vi "datatojson.vi"() -> (3 "json":string[](array[string]))   [LabVIEW 2022 SP3, in "工况数据上传.lvlib"]
panel:
  out "data":T1={"time"="2021-05-08 14-02-02", "data"={"ups"={"ups"={"input_voltage"=0.0, "input_frequency"=0.0, "output_voltage"=0.0, "output_current"=0.0, "output_frequency"=0.0, "output_active_power"=0.0, "output_apparent_power"=0.0, "load_rate"=0.0, "cabinet_temperature"=0.0, "battery_voltage"=0.0, "remaining_battery_capacity"=0.0, "power_on_status"="", "power_supply_mode"="", "fault"=FALSE, "battery_low_voltage"=FALSE, "mains_supply_abnormality"=FALSE}, "启用"=FALSE}, "air_conditioner"={"air_conditioner"={"cabinet_temperature"=0.0, "air_supply_temperature"=0.0, "voltage"=0.0, "current"=0.0, "compressor_status"="", "Internal_fan_status"="", "external_fan_status"="", "heating_state"="", "refrigeration_state"=FALSE, "high_temperature_alarm"=FALSE, "low_temperature_alarm"=FALSE, "heater_fault"=FALSE, "temperature_sensor_fault"=FALSE, "high_voltage_alarm"=FALSE, "low_voltage_alarm"=FALSE, "refrigeration_start_point"=0.0, "refrigeration_sensitive_point"=0.0, "heating_start_point"=0.0, "heating_sensitive_point"=0.0, "high_temperature_alarm_point"=0.0, "low_temperature_alarm_point"=0.0}, "启用"=FALSE}, "smoke_sensor"={"smoke_sensor"={"trigger_alarm"=FALSE}, "启用"=FALSE}, "water_immersion_sensor"={"water_immersion_sensor"={"trigger_alarm"=FALSE}, "启用"=FALSE}, "temperature_and_humidity_sensor"={"temperature_and_humidity_sensor"={"current_temperature"=0.0, "current_humidity"=0.0, "room_temperature_alarm"=FALSE, "humidity_alarm"=FALSE}, "启用"=FALSE}, "gps"={"gps"={"current_longitude"=0.0, "current_latitude"=0.0, "launch_longitude"=0.0, "launch_latitude"=0.0, "shift_alarm"=FALSE}, "启用"=FALSE}, "solar_controller"={"solar_controller"={"array_voltage"=0.0, "array_current"=0.0, "generating_power"=0.0, "battery_voltage"=0.0, "battery_current"=0.0, "ceiling_voltage"=0.0, "minimum_voltage"=0.0, "battery_temperature"=0.0, "remaining_battery_capacity"=0.0, "load_voltage"=0.0, "load_current"=0.0, "load_power"=0.0, "equipment_temperature"=0.0, "accumulated_electricity_consumption_of_the_day"=0.0, "accumulated_electricity_consumption_of_the_current_month"=0.0, "accumulated_electricity_consumption_in_the_current_year"=0.0, "total_accumulated_power_consumption"=0.0, "accumulated_charging_capacity_of_the_day"=0.0, "accumulated_charging_amount_of_the_current_month"=0.0, "accumulated_charging_capacity_of_the_current_year"=0.0, "total_cumulative_charge"=0.0}, "启用"=FALSE}, "solar_controller_2"={"solar_controller_2"={"array_voltage"=0.0, "array_current"=0.0, "generating_power"=0.0, "battery_voltage"=0.0, "battery_current"=0.0, "ceiling_voltage"=0.0, "minimum_voltage"=0.0, "battery_temperature"=0.0, "remaining_battery_capacity"=0.0, "load_voltage"=0.0, "load_current"=0.0, "load_power"=0.0, "equipment_temperature"=0.0, "accumulated_electricity_consumption_of_the_day"=0.0, "accumulated_electricity_consumption_of_the_current_month"=0.0, "accumulated_electricity_consumption_in_the_current_year"=0.0, "total_accumulated_power_consumption"=0.0, "accumulated_charging_capacity_of_the_day"=0.0, "accumulated_charging_amount_of_the_current_month"=0.0, "accumulated_charging_capacity_of_the_current_year"=0.0, "total_cumulative_charge"=0.0}, "启用"=FALSE}, "NH3"={"NH3"={"F0"=0.0, "F1"=0.0, "syringe_temperature"=0.0, "alarm_step"=0.0, "X0"=0.0}, "启用"=FALSE}, "TP"={"TP"={"F0"=0.0, "F1"=0.0, "F2"=0.0, "F3"=0.0, "digestion_temperature"=0.0, "constant_temperature"=0.0, "syringe_temperature"=0.0, "alarm_step"=0.0, "X0"=0.0}, "启用"=FALSE}, "TN"={"TN"={"F0"=0.0, "F1"=0.0, "F2"=0.0, "F3"=0.0, "F4"=0.0, "F5"=0.0, "F6"=0.0, "F7"=0.0, "digestion_temperature"=0.0, "constant_temperature"=0.0, "syringe_temperature"=0.0, "alarm_step"=0.0, "X0"=0.0}, "启用"=FALSE}, "CODMn"={"CODMn"={"temperature_curve"=[], "titration_curve"=[], "F0"=0.0, "F1"=0.0, "F2"=0.0, "F3"=0.0, "F4"=0.0, "F5"=0.0, "A"=0.0, "B"=0.0, "K"=0.0}, "启用"=FALSE}, "CODCr"={"CODCr"={"temperature_curve"=[], "F0"=0.0, "F1"=0.0, "reagent_sensor"=0.0}, "启用"=FALSE}}} {"data"."air_conditioner"."air_conditioner"."current" format="%#.2g"}
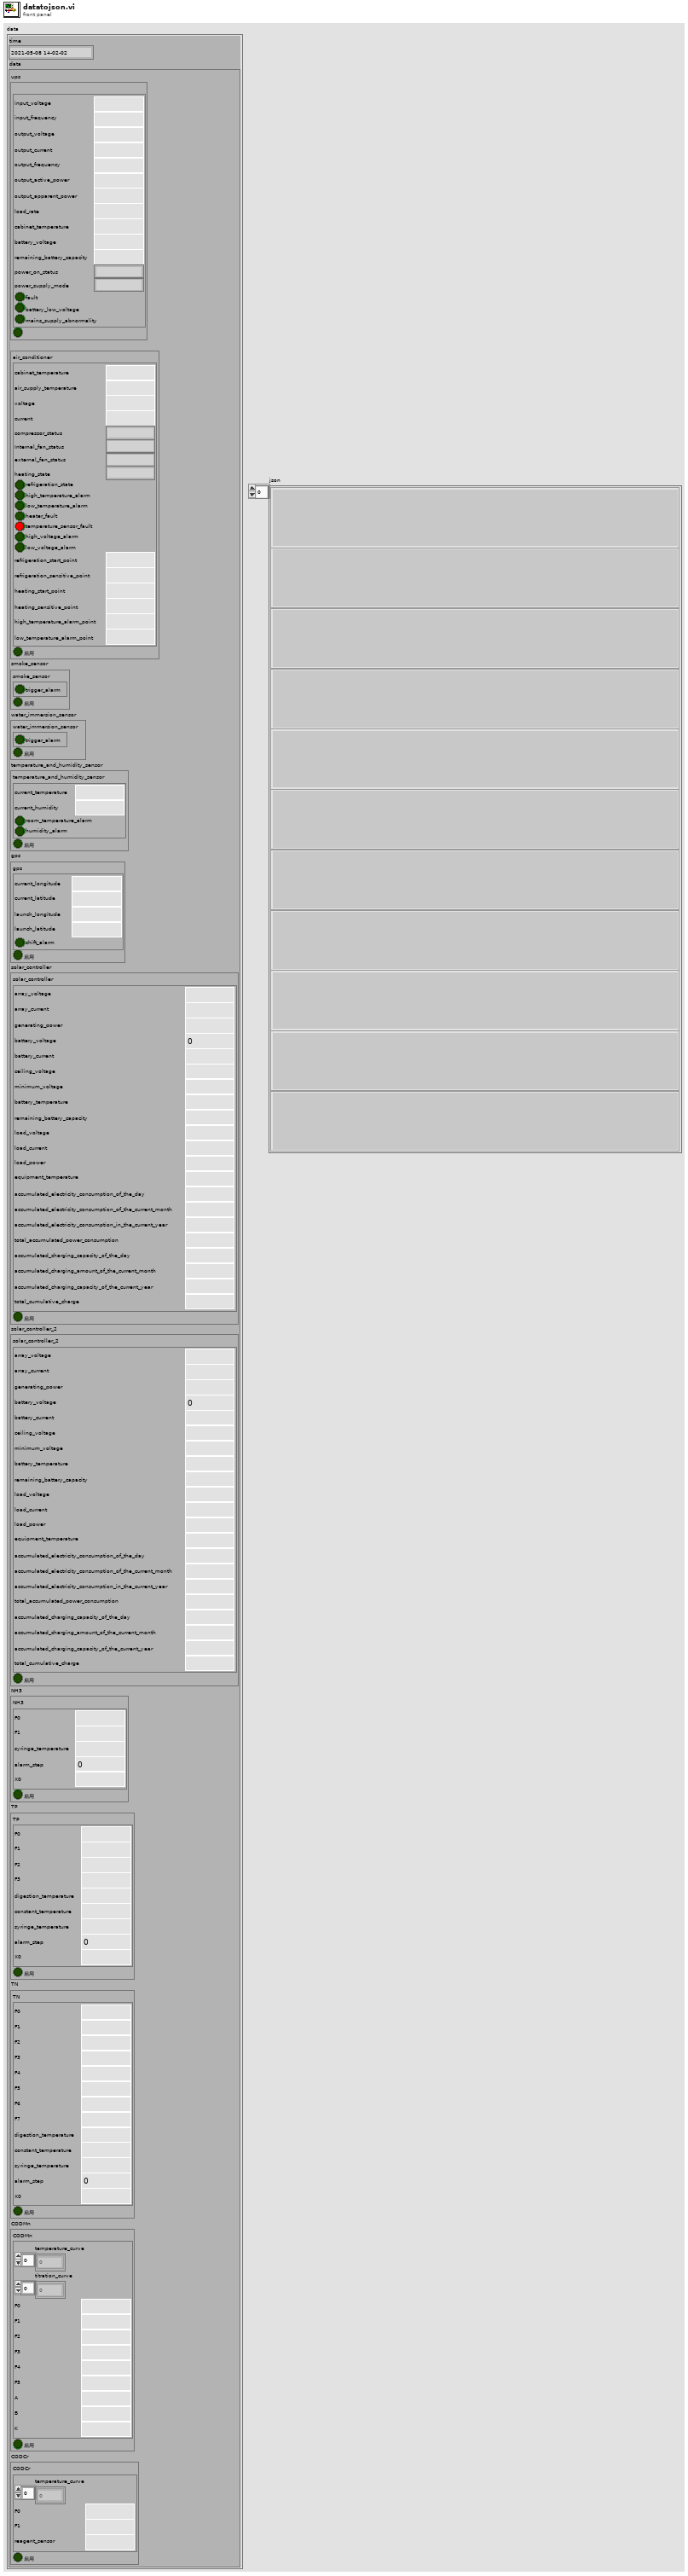
[diagram p1: front panel]
types:
  T1 = typedef "工况数据.ctl" = cluster{"time":string, "data":cluster{"ups":cluster{"ups":cluster{"input_voltage":ext, "input_frequency":ext, "output_voltage":ext, "output_current":ext, "output_frequency":ext, "output_active_power":ext, "output_apparent_power":ext, "load_rate":ext, "cabinet_temperature":ext, "battery_voltage":ext, "remaining_battery_capacity":ext, "power_on_status":string, "power_supply_mode":string, "fault":bool, "battery_low_voltage":bool, "mains_supply_abnormality":bool}, "启用":bool}, "air_conditioner":cluster{"air_conditioner":cluster{"cabinet_temperature":ext, "air_supply_temperature":ext, "voltage":ext, "current":ext, "compressor_status":string, "Internal_fan_status":string, "external_fan_status":string, "heating_state":string, "refrigeration_state":bool, "high_temperature_alarm":bool, "low_temperature_alarm":bool, "heater_fault":bool, "temperature_sensor_fault":bool, "high_voltage_alarm":bool, "low_voltage_alarm":bool, "refrigeration_start_point":ext, "refrigeration_sensitive_point":ext, "heating_start_point":ext, "heating_sensitive_point":ext, "high_temperature_alarm_point":ext, "low_temperature_alarm_point":ext}, "启用":bool}, "smoke_sensor":cluster{"smoke_sensor":cluster{"trigger_alarm":bool}, "启用":bool}, "water_immersion_sensor":cluster{"water_immersion_sensor":cluster{"trigger_alarm":bool}, "启用":bool}, "temperature_and_humidity_sensor":cluster{"temperature_and_humidity_sensor":cluster{"current_temperature":ext, "current_humidity":ext, "room_temperature_alarm":bool, "humidity_alarm":bool}, "启用":bool}, "gps":cluster{"gps":cluster{"current_longitude":ext, "current_latitude":ext, "launch_longitude":ext, "launch_latitude":ext, "shift_alarm":bool}, "启用":bool}, "solar_controller":cluster{"solar_controller":cluster{"array_voltage":ext, "array_current":ext, "generating_power":ext, "battery_voltage":dbl, "battery_current":ext, "ceiling_voltage":ext, "minimum_voltage":ext, "battery_temperature":ext, "remaining_battery_capacity":ext, "load_voltage":ext, "load_current":ext, "load_power":ext, "equipment_temperature":ext, "accumulated_electricity_consumption_of_the_day":ext, "accumulated_electricity_consumption_of_the_current_month":ext, "accumulated_electricity_consumption_in_the_current_year":ext, "total_accumulated_power_consumption":ext, "accumulated_charging_capacity_of_the_day":ext, "accumulated_charging_amount_of_the_current_month":ext, "accumulated_charging_capacity_of_the_current_year":ext, "total_cumulative_charge":ext}, "启用":bool}, "solar_controller_2":cluster{"solar_controller_2":cluster{"array_voltage":ext, "array_current":ext, "generating_power":ext, "battery_voltage":dbl, "battery_current":ext, "ceiling_voltage":ext, "minimum_voltage":ext, "battery_temperature":ext, "remaining_battery_capacity":ext, "load_voltage":ext, "load_current":ext, "load_power":ext, "equipment_temperature":ext, "accumulated_electricity_consumption_of_the_day":ext, "accumulated_electricity_consumption_of_the_current_month":ext, "accumulated_electricity_consumption_in_the_current_year":ext, "total_accumulated_power_consumption":ext, "accumulated_charging_capacity_of_the_day":ext, "accumulated_charging_amount_of_the_current_month":ext, "accumulated_charging_capacity_of_the_current_year":ext, "total_cumulative_charge":ext}, "启用":bool}, "NH3":cluster{"NH3":cluster{"F0":ext, "F1":ext, "syringe_temperature":ext, "alarm_step":dbl, "X0":ext}, "启用":bool}, "TP":cluster{"TP":cluster{"F0":ext, "F1":ext, "F2":ext, "F3":ext, "digestion_temperature":ext, "constant_temperature":ext, "syringe_temperature":ext, "alarm_step":dbl, "X0":ext}, "启用":bool}, "TN":cluster{"TN":cluster{"F0":ext, "F1":ext, "F2":ext, "F3":ext, "F4":ext, "F5":ext, "F6":ext, "F7":ext, "digestion_temperature":ext, "constant_temperature":ext, "syringe_temperature":ext, "alarm_step":dbl, "X0":ext}, "启用":bool}, "CODMn":cluster{"CODMn":cluster{"temperature_curve":ext[], "titration_curve":ext[], "F0":ext, "F1":ext, "F2":ext, "F3":ext, "F4":ext, "F5":ext, "A":ext, "B":ext, "K":ext}, "启用":bool}, "CODCr":cluster{"CODCr":cluster{"temperature_curve":ext[], "F0":ext, "F1":ext, "reagent_sensor":ext}, "启用":bool}}}
  T2 = cluster{"ups":cluster{"ups":cluster{"input_voltage":ext, "input_frequency":ext, "output_voltage":ext, "output_current":ext, "output_frequency":ext, "output_active_power":ext, "output_apparent_power":ext, "load_rate":ext, "cabinet_temperature":ext, "battery_voltage":ext, "remaining_battery_capacity":ext, "power_on_status":string, "power_supply_mode":string, "fault":bool, "battery_low_voltage":bool, "mains_supply_abnormality":bool}, "启用":bool}, "air_conditioner":cluster{"air_conditioner":cluster{"cabinet_temperature":ext, "air_supply_temperature":ext, "voltage":ext, "current":ext, "compressor_status":string, "Internal_fan_status":string, "external_fan_status":string, "heating_state":string, "refrigeration_state":bool, "high_temperature_alarm":bool, "low_temperature_alarm":bool, "heater_fault":bool, "temperature_sensor_fault":bool, "high_voltage_alarm":bool, "low_voltage_alarm":bool, "refrigeration_start_point":ext, "refrigeration_sensitive_point":ext, "heating_start_point":ext, "heating_sensitive_point":ext, "high_temperature_alarm_point":ext, "low_temperature_alarm_point":ext}, "启用":bool}, "smoke_sensor":cluster{"smoke_sensor":cluster{"trigger_alarm":bool}, "启用":bool}, "water_immersion_sensor":cluster{"water_immersion_sensor":cluster{"trigger_alarm":bool}, "启用":bool}, "temperature_and_humidity_sensor":cluster{"temperature_and_humidity_sensor":cluster{"current_temperature":ext, "current_humidity":ext, "room_temperature_alarm":bool, "humidity_alarm":bool}, "启用":bool}, "gps":cluster{"gps":cluster{"current_longitude":ext, "current_latitude":ext, "launch_longitude":ext, "launch_latitude":ext, "shift_alarm":bool}, "启用":bool}, "solar_controller":cluster{"solar_controller":cluster{"array_voltage":ext, "array_current":ext, "generating_power":ext, "battery_voltage":dbl, "battery_current":ext, "ceiling_voltage":ext, "minimum_voltage":ext, "battery_temperature":ext, "remaining_battery_capacity":ext, "load_voltage":ext, "load_current":ext, "load_power":ext, "equipment_temperature":ext, "accumulated_electricity_consumption_of_the_day":ext, "accumulated_electricity_consumption_of_the_current_month":ext, "accumulated_electricity_consumption_in_the_current_year":ext, "total_accumulated_power_consumption":ext, "accumulated_charging_capacity_of_the_day":ext, "accumulated_charging_amount_of_the_current_month":ext, "accumulated_charging_capacity_of_the_current_year":ext, "total_cumulative_charge":ext}, "启用":bool}, "solar_controller_2":cluster{"solar_controller_2":cluster{"array_voltage":ext, "array_current":ext, "generating_power":ext, "battery_voltage":dbl, "battery_current":ext, "ceiling_voltage":ext, "minimum_voltage":ext, "battery_temperature":ext, "remaining_battery_capacity":ext, "load_voltage":ext, "load_current":ext, "load_power":ext, "equipment_temperature":ext, "accumulated_electricity_consumption_of_the_day":ext, "accumulated_electricity_consumption_of_the_current_month":ext, "accumulated_electricity_consumption_in_the_current_year":ext, "total_accumulated_power_consumption":ext, "accumulated_charging_capacity_of_the_day":ext, "accumulated_charging_amount_of_the_current_month":ext, "accumulated_charging_capacity_of_the_current_year":ext, "total_cumulative_charge":ext}, "启用":bool}, "NH3":cluster{"NH3":cluster{"F0":ext, "F1":ext, "syringe_temperature":ext, "alarm_step":dbl, "X0":ext}, "启用":bool}, "TP":cluster{"TP":cluster{"F0":ext, "F1":ext, "F2":ext, "F3":ext, "digestion_temperature":ext, "constant_temperature":ext, "syringe_temperature":ext, "alarm_step":dbl, "X0":ext}, "启用":bool}, "TN":cluster{"TN":cluster{"F0":ext, "F1":ext, "F2":ext, "F3":ext, "F4":ext, "F5":ext, "F6":ext, "F7":ext, "digestion_temperature":ext, "constant_temperature":ext, "syringe_temperature":ext, "alarm_step":dbl, "X0":ext}, "启用":bool}, "CODMn":cluster{"CODMn":cluster{"temperature_curve":ext[], "titration_curve":ext[], "F0":ext, "F1":ext, "F2":ext, "F3":ext, "F4":ext, "F5":ext, "A":ext, "B":ext, "K":ext}, "启用":bool}, "CODCr":cluster{"CODCr":cluster{"temperature_curve":ext[], "F0":ext, "F1":ext, "reagent_sensor":ext}, "启用":bool}}
  T3 = cluster{"ups":cluster{"input_voltage":ext, "input_frequency":ext, "output_voltage":ext, "output_current":ext, "output_frequency":ext, "output_active_power":ext, "output_apparent_power":ext, "load_rate":ext, "cabinet_temperature":ext, "battery_voltage":ext, "remaining_battery_capacity":ext, "power_on_status":string, "power_supply_mode":string, "fault":bool, "battery_low_voltage":bool, "mains_supply_abnormality":bool}, "启用":bool}
  T4 = cluster{"air_conditioner":cluster{"cabinet_temperature":ext, "air_supply_temperature":ext, "voltage":ext, "current":ext, "compressor_status":string, "Internal_fan_status":string, "external_fan_status":string, "heating_state":string, "refrigeration_state":bool, "high_temperature_alarm":bool, "low_temperature_alarm":bool, "heater_fault":bool, "temperature_sensor_fault":bool, "high_voltage_alarm":bool, "low_voltage_alarm":bool, "refrigeration_start_point":ext, "refrigeration_sensitive_point":ext, "heating_start_point":ext, "heating_sensitive_point":ext, "high_temperature_alarm_point":ext, "low_temperature_alarm_point":ext}, "启用":bool}
  T5 = cluster{"smoke_sensor":cluster{"trigger_alarm":bool}, "启用":bool}
  T6 = cluster{"water_immersion_sensor":cluster{"trigger_alarm":bool}, "启用":bool}
  T7 = cluster{"temperature_and_humidity_sensor":cluster{"current_temperature":ext, "current_humidity":ext, "room_temperature_alarm":bool, "humidity_alarm":bool}, "启用":bool}
  T8 = cluster{"gps":cluster{"current_longitude":ext, "current_latitude":ext, "launch_longitude":ext, "launch_latitude":ext, "shift_alarm":bool}, "启用":bool}
  T9 = cluster{"solar_controller":cluster{"array_voltage":ext, "array_current":ext, "generating_power":ext, "battery_voltage":dbl, "battery_current":ext, "ceiling_voltage":ext, "minimum_voltage":ext, "battery_temperature":ext, "remaining_battery_capacity":ext, "load_voltage":ext, "load_current":ext, "load_power":ext, "equipment_temperature":ext, "accumulated_electricity_consumption_of_the_day":ext, "accumulated_electricity_consumption_of_the_current_month":ext, "accumulated_electricity_consumption_in_the_current_year":ext, "total_accumulated_power_consumption":ext, "accumulated_charging_capacity_of_the_day":ext, "accumulated_charging_amount_of_the_current_month":ext, "accumulated_charging_capacity_of_the_current_year":ext, "total_cumulative_charge":ext}, "启用":bool}
  T10 = cluster{"solar_controller_2":cluster{"array_voltage":ext, "array_current":ext, "generating_power":ext, "battery_voltage":dbl, "battery_current":ext, "ceiling_voltage":ext, "minimum_voltage":ext, "battery_temperature":ext, "remaining_battery_capacity":ext, "load_voltage":ext, "load_current":ext, "load_power":ext, "equipment_temperature":ext, "accumulated_electricity_consumption_of_the_day":ext, "accumulated_electricity_consumption_of_the_current_month":ext, "accumulated_electricity_consumption_in_the_current_year":ext, "total_accumulated_power_consumption":ext, "accumulated_charging_capacity_of_the_day":ext, "accumulated_charging_amount_of_the_current_month":ext, "accumulated_charging_capacity_of_the_current_year":ext, "total_cumulative_charge":ext}, "启用":bool}
  T11 = cluster{"NH3":cluster{"F0":ext, "F1":ext, "syringe_temperature":ext, "alarm_step":dbl, "X0":ext}, "启用":bool}
  T12 = cluster{"TP":cluster{"F0":ext, "F1":ext, "F2":ext, "F3":ext, "digestion_temperature":ext, "constant_temperature":ext, "syringe_temperature":ext, "alarm_step":dbl, "X0":ext}, "启用":bool}
  T13 = cluster{"TN":cluster{"F0":ext, "F1":ext, "F2":ext, "F3":ext, "F4":ext, "F5":ext, "F6":ext, "F7":ext, "digestion_temperature":ext, "constant_temperature":ext, "syringe_temperature":ext, "alarm_step":dbl, "X0":ext}, "启用":bool}
  T14 = cluster{"CODMn":cluster{"temperature_curve":ext[], "titration_curve":ext[], "F0":ext, "F1":ext, "F2":ext, "F3":ext, "F4":ext, "F5":ext, "A":ext, "B":ext, "K":ext}, "启用":bool}
  T15 = cluster{"CODCr":cluster{"temperature_curve":ext[], "F0":ext, "F1":ext, "reagent_sensor":ext}, "启用":bool}
  T16 = cluster{"current_temperature":ext, "current_humidity":ext, "room_temperature_alarm":bool, "humidity_alarm":bool}
  T17 = cluster{"array_voltage":ext, "array_current":ext, "generating_power":ext, "battery_voltage":dbl, "battery_current":ext, "ceiling_voltage":ext, "minimum_voltage":ext, "battery_temperature":ext, "remaining_battery_capacity":ext, "load_voltage":ext, "load_current":ext, "load_power":ext, "equipment_temperature":ext, "accumulated_electricity_consumption_of_the_day":ext, "accumulated_electricity_consumption_of_the_current_month":ext, "accumulated_electricity_consumption_in_the_current_year":ext, "total_accumulated_power_consumption":ext, "accumulated_charging_capacity_of_the_day":ext, "accumulated_charging_amount_of_the_current_month":ext, "accumulated_charging_capacity_of_the_current_year":ext, "total_cumulative_charge":ext}
  T18 = cluster{"cabinet_temperature":ext, "air_supply_temperature":ext, "voltage":ext, "current":ext, "compressor_status":string, "Internal_fan_status":string, "external_fan_status":string, "heating_state":string, "refrigeration_state":bool, "high_temperature_alarm":bool, "low_temperature_alarm":bool, "heater_fault":bool, "temperature_sensor_fault":bool, "high_voltage_alarm":bool, "low_voltage_alarm":bool, "refrigeration_start_point":ext, "refrigeration_sensitive_point":ext, "heating_start_point":ext, "heating_sensitive_point":ext, "high_temperature_alarm_point":ext, "low_temperature_alarm_point":ext}
  T19 = cluster{"temperature_curve":ext[], "titration_curve":ext[], "F0":ext, "F1":ext, "F2":ext, "F3":ext, "F4":ext, "F5":ext, "A":ext, "B":ext, "K":ext}
  T20 = cluster{"temperature_curve":ext[], "F0":ext, "F1":ext, "reagent_sensor":ext}
  T21 = cluster{"F0":ext, "F1":ext, "syringe_temperature":ext, "alarm_step":dbl, "X0":ext}
  T22 = cluster{"input_voltage":ext, "input_frequency":ext, "output_voltage":ext, "output_current":ext, "output_frequency":ext, "output_active_power":ext, "output_apparent_power":ext, "load_rate":ext, "cabinet_temperature":ext, "battery_voltage":ext, "remaining_battery_capacity":ext, "power_on_status":string, "power_supply_mode":string, "fault":bool, "battery_low_voltage":bool, "mains_supply_abnormality":bool}
  T23 = cluster{"current_longitude":ext, "current_latitude":ext, "launch_longitude":ext, "launch_latitude":ext, "shift_alarm":bool}
  T24 = cluster{"F0":ext, "F1":ext, "F2":ext, "F3":ext, "digestion_temperature":ext, "constant_temperature":ext, "syringe_temperature":ext, "alarm_step":dbl, "X0":ext}
  T25 = cluster{"F0":ext, "F1":ext, "F2":ext, "F3":ext, "F4":ext, "F5":ext, "F6":ext, "F7":ext, "digestion_temperature":ext, "constant_temperature":ext, "syringe_temperature":ext, "alarm_step":dbl, "X0":ext}
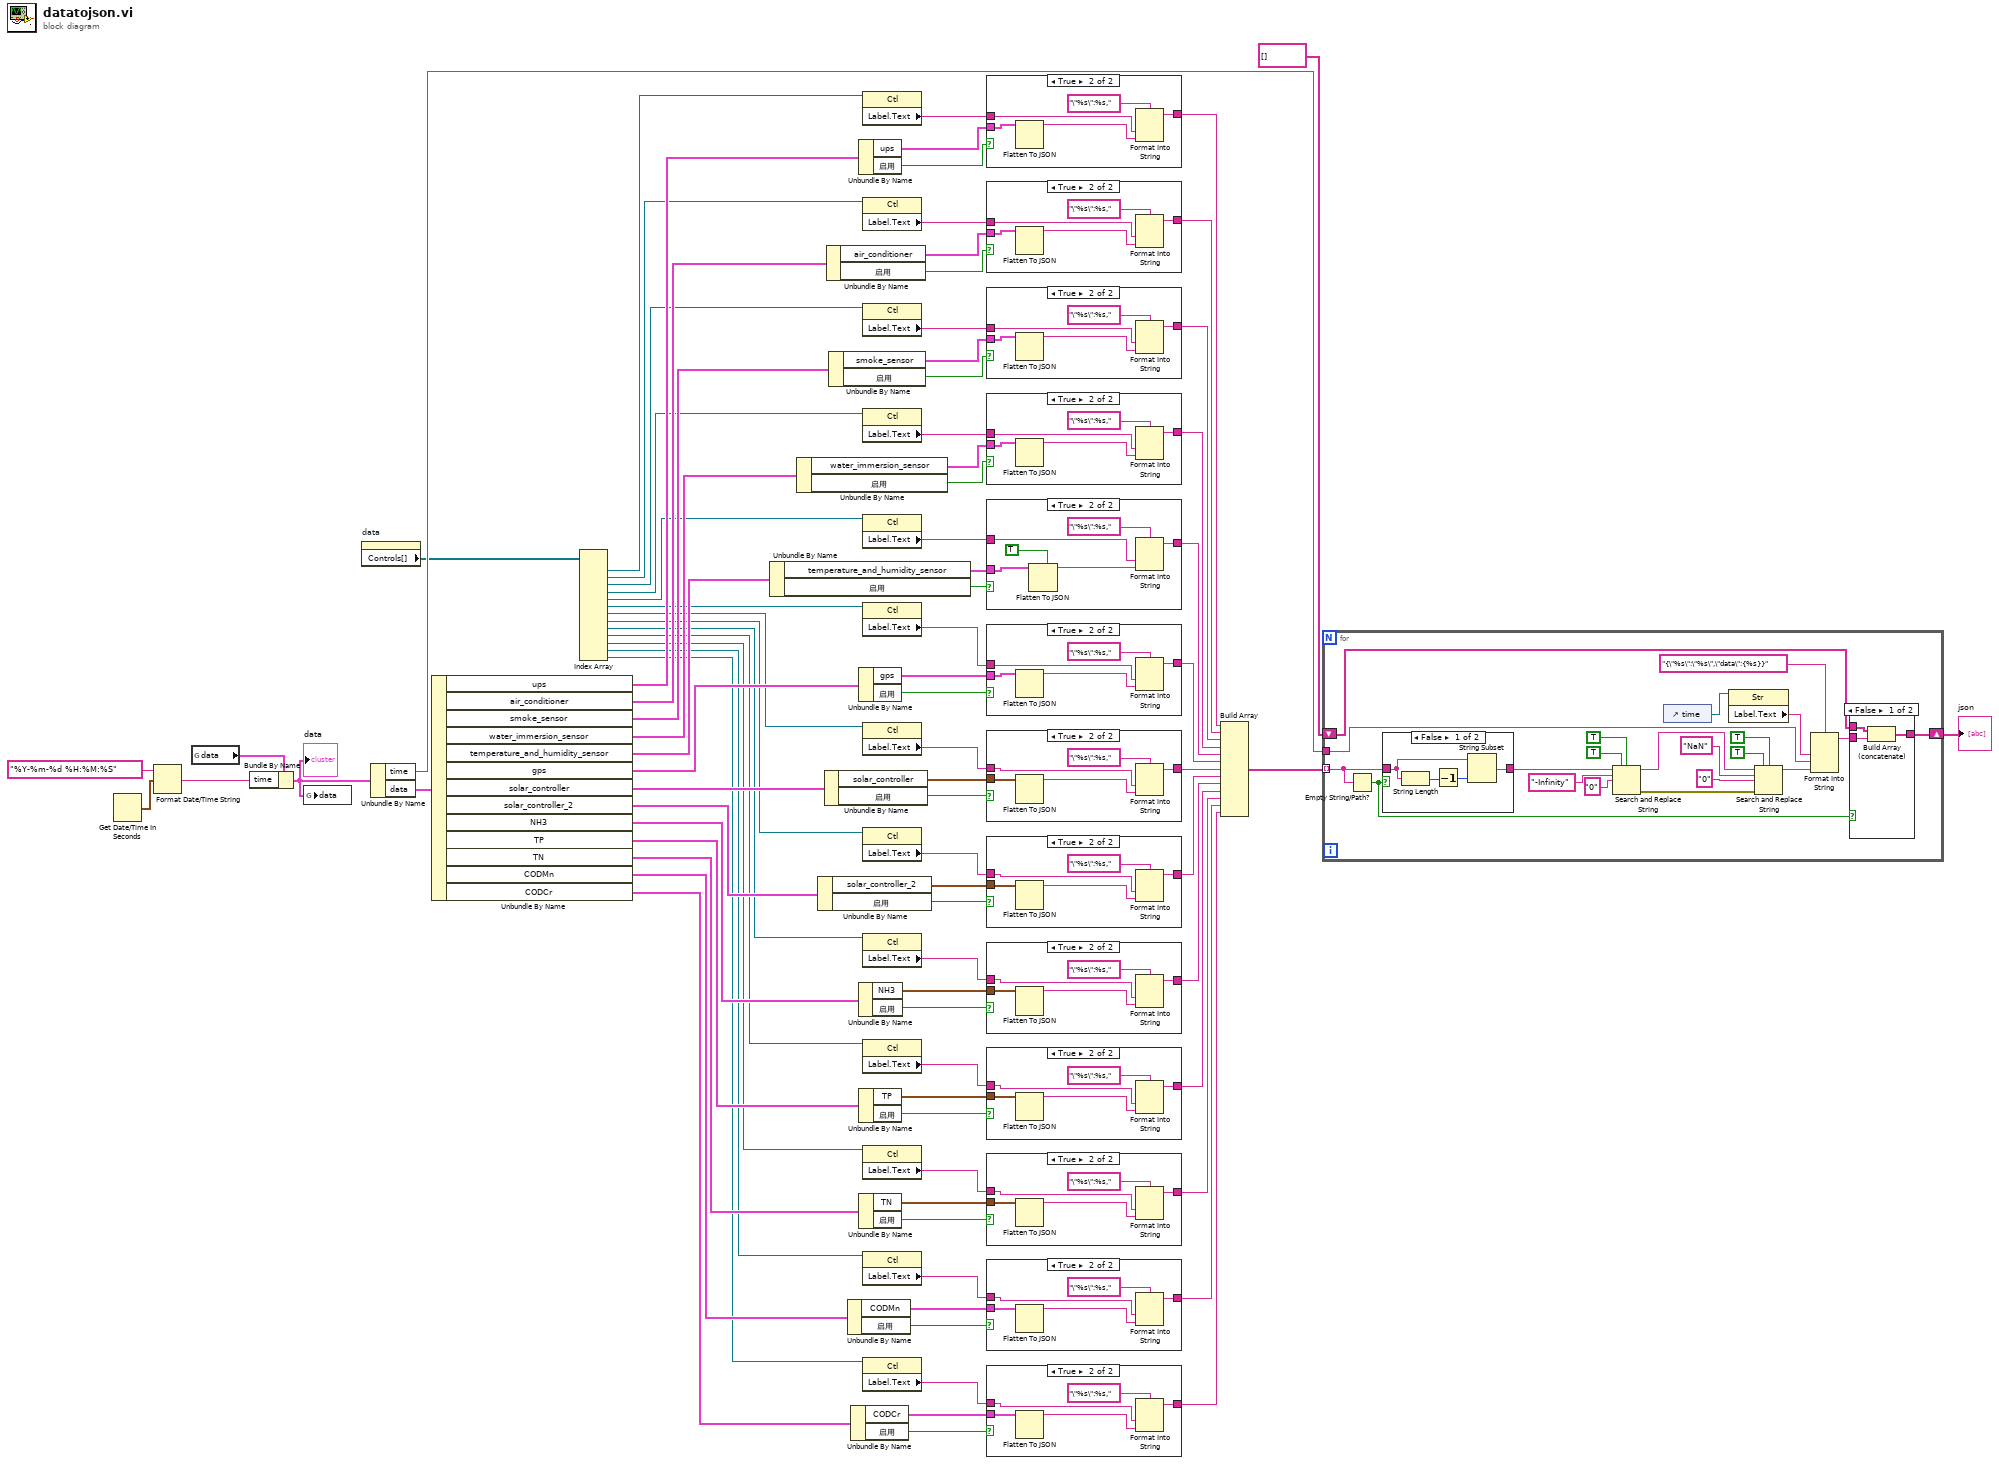
[diagram p0: block diagram]
diagram:
  n1 = Get Date/Time In Seconds() -> (seconds since 1Jan1904=w48:timestamp)
  n2 = Format Date/Time String(time format string (%c)="%Y-%m-%d %H:%M:%S" ("时间格式字符串(%c)"), seconds (now)=w48) -> (date/time string=w46:string)  [unwired: 1 in]
  n3 = global read "工况数据接口全局.vi" "data"() -> (w47:T1)
  n4 = Bundle By Name(cluster=w47, "time"=w46) -> (w42:T1)
  "data" <- w42
  n5 = global write "工况数据接口全局.vi" "data"(w42) -> ()
  n6 = property on="data" class="Clust (strict)"() -> ("Controls[]"=w43:refnum<vi>[])  [unwired: 2 in, 2 out]
  n7 = Unbundle By Name(w42) -> ("time"=w45:string, "data"=w44:T2)
  n8 = Unbundle By Name(w44) -> ("ups"=w89:T3, "air_conditioner"=w84:T4, "smoke_sensor"=w75:T5, "water_immersion_sensor"=w70:T6, "temperature_and_humidity_sensor"=w66:T7, "gps"=w61:T8, "solar_controller"=w55:T9, "solar_controller_2"=w50:T10, "NH3"=w27:T11, "TP"=w12:T12, "TN"=w10:T13, "CODMn"=w8:T14, "CODCr"=w6:T15)
  n9 = Index Array(array=w43) -> (element #1=w87:refnum<vi>, element #2=w81:refnum<vi>, element #3=w76:refnum<vi>, element #4=w71:refnum<vi>, element #5=w65:refnum<vi>, element #6=w60:refnum<vi>, element #7=w56:refnum<vi>, element #8=w51:refnum<vi>, element #9=w26:refnum<vi>, element #10=w13:refnum<vi>, element #11=w11:refnum<vi>, element #12=w9:refnum<vi>, element #13=w7:refnum<vi>)  [unwired: 13 in]
  n10 = Unbundle By Name(w66) -> ("temperature_and_humidity_sensor"=w68:T16, "启用"=w69:bool)
  n11 = Unbundle By Name(w70) -> ("water_immersion_sensor"=w73:cluster{"trigger_alarm":bool}, "启用"=w74:bool)
  n12 = Unbundle By Name(w50) -> ("solar_controller_2"=w53:T17, "启用"=w54:bool)
  n13 = Unbundle By Name(w55) -> ("solar_controller"=w58:T17, "启用"=w59:bool)
  n14 = Unbundle By Name(w84) -> ("air_conditioner"=w82:T18, "启用"=w83:bool)
  n15 = Unbundle By Name(w75) -> ("smoke_sensor"=w78:cluster{"trigger_alarm":bool}, "启用"=w77:bool)
  n16 = Unbundle By Name(w8) -> ("CODMn"=w15:T19, "启用"=w14:bool)
  n17 = Unbundle By Name(w6) -> ("CODCr"=w18:T20, "启用"=w19:bool)
  n18 = Unbundle By Name(w27) -> ("NH3"=w29:T21, "启用"=w28:bool)
  n19 = Unbundle By Name(w89) -> ("ups"=w88:T22, "启用"=w85:bool)
  n20 = Unbundle By Name(w61) -> ("gps"=w63:T23, "启用"=w64:bool)
  n21 = Unbundle By Name(w12) -> ("TP"=w24:T24, "启用"=w25:bool)
  n22 = Unbundle By Name(w10) -> ("TN"=w21:T25, "启用"=w20:bool)
  n23 = property class="Ctl"(reference=w87) -> ("Label.Text"=w86:string)  [unwired: 1 in, 2 out]
  n24 = property class="Ctl"(reference=w81) -> ("Label.Text"=w80:string)  [unwired: 1 in, 2 out]
  n25 = property class="Ctl"(reference=w76) -> ("Label.Text"=w79:string)  [unwired: 1 in, 2 out]
  n26 = property class="Ctl"(reference=w71) -> ("Label.Text"=w72:string)  [unwired: 1 in, 2 out]
  n27 = property class="Ctl"(reference=w65) -> ("Label.Text"=w67:string)  [unwired: 1 in, 2 out]
  n28 = property class="Ctl"(reference=w60) -> ("Label.Text"=w62:string)  [unwired: 1 in, 2 out]
  n29 = property class="Ctl"(reference=w56) -> ("Label.Text"=w57:string)  [unwired: 1 in, 2 out]
  n30 = property class="Ctl"(reference=w51) -> ("Label.Text"=w52:string)  [unwired: 1 in, 2 out]
  n31 = property class="Ctl"(reference=w26) -> ("Label.Text"=w30:string)  [unwired: 1 in, 2 out]
  n32 = property class="Ctl"(reference=w13) -> ("Label.Text"=w23:string)  [unwired: 1 in, 2 out]
  n33 = property class="Ctl"(reference=w11) -> ("Label.Text"=w22:string)  [unwired: 1 in, 2 out]
  n34 = property class="Ctl"(reference=w9) -> ("Label.Text"=w16:string)  [unwired: 1 in, 2 out]
  n35 = property class="Ctl"(reference=w7) -> ("Label.Text"=w17:string)  [unwired: 1 in, 2 out]
  n36 = case shown="True" w85 {
    tunnel: w88 -> [_ w94]
    tunnel: w86 -> [_ w92]
    tunnel: [_ w91] -> w41
    frame False {
    }
    frame True {
      n37 = Flatten To JSON(anything=w94) -> (JSON string=w90:string)  [unwired: 2 in, 1 out]
      n38 = Format Into String(format string="\"%s\":%s," ("格式字符串"), w92, w90) -> (resulting string=w91:string)  [unwired: 2 in, 1 out]
    }
  }
  n39 = case shown="True" w83 {
    tunnel: w82 -> [_ w99]
    tunnel: w80 -> [_ w97]
    tunnel: [_ w96] -> w40
    frame False {
    }
    frame True {
      n40 = Flatten To JSON(anything=w99) -> (JSON string=w95:string)  [unwired: 2 in, 1 out]
      n41 = Format Into String(format string="\"%s\":%s," ("格式字符串"), w97, w95) -> (resulting string=w96:string)  [unwired: 2 in, 1 out]
    }
  }
  n42 = case shown="True" w77 {
    tunnel: w78 -> [_ w104]
    tunnel: w79 -> [_ w102]
    tunnel: [_ w101] -> w39
    frame False {
    }
    frame True {
      n43 = Flatten To JSON(anything=w104) -> (JSON string=w100:string)  [unwired: 2 in, 1 out]
      n44 = Format Into String(format string="\"%s\":%s," ("格式字符串"), w102, w100) -> (resulting string=w101:string)  [unwired: 2 in, 1 out]
    }
  }
  n45 = case shown="True" w74 {
    tunnel: w73 -> [_ w109]
    tunnel: w72 -> [_ w107]
    tunnel: [_ w106] -> w38
    frame False {
    }
    frame True {
      n46 = Flatten To JSON(anything=w109) -> (JSON string=w105:string)  [unwired: 2 in, 1 out]
      n47 = Format Into String(format string="\"%s\":%s," ("格式字符串"), w107, w105) -> (resulting string=w106:string)  [unwired: 2 in, 1 out]
    }
  }
  n48 = case shown="True" w69 {
    tunnel: w68 -> [_ w115]
    tunnel: w67 -> [_ w113]
    tunnel: [_ w112] -> w37
    frame False {
    }
    frame True {
      n49 = Flatten To JSON(enable LabVIEW extensions? (T)=TRUE ("启用LabVIEW扩展？(T)"), anything=w115) -> (JSON string=w111:string)  [unwired: 1 in, 1 out]
      n50 = Format Into String(format string="\"%s\":%s," ("格式字符串"), w113, w111) -> (resulting string=w112:string)  [unwired: 2 in, 1 out]
    }
  }
  n51 = case shown="True" w64 {
    tunnel: w63 -> [_ w120]
    tunnel: w62 -> [_ w118]
    tunnel: [_ w117] -> w36
    frame False {
    }
    frame True {
      n52 = Flatten To JSON(anything=w120) -> (JSON string=w116:string)  [unwired: 2 in, 1 out]
      n53 = Format Into String(format string="\"%s\":%s," ("格式字符串"), w118, w116) -> (resulting string=w117:string)  [unwired: 2 in, 1 out]
    }
  }
  n54 = case shown="True" w59 {
    tunnel: w58 -> [_ w125]
    tunnel: w57 -> [_ w123]
    tunnel: [_ w122] -> w35
    frame False {
    }
    frame True {
      n55 = Flatten To JSON(anything=w125) -> (JSON string=w121:string)  [unwired: 2 in, 1 out]
      n56 = Format Into String(format string="\"%s\":%s," ("格式字符串"), w123, w121) -> (resulting string=w122:string)  [unwired: 2 in, 1 out]
    }
  }
  n57 = case shown="True" w54 {
    tunnel: w53 -> [_ w130]
    tunnel: w52 -> [_ w128]
    tunnel: [_ w127] -> w34
    frame False {
    }
    frame True {
      n58 = Flatten To JSON(anything=w130) -> (JSON string=w126:string)  [unwired: 2 in, 1 out]
      n59 = Format Into String(format string="\"%s\":%s," ("格式字符串"), w128, w126) -> (resulting string=w127:string)  [unwired: 2 in, 1 out]
    }
  }
  n60 = case shown="True" w28 {
    tunnel: w29 -> [_ w135]
    tunnel: w30 -> [_ w133]
    tunnel: [_ w132] -> w5
    frame False {
    }
    frame True {
      n61 = Flatten To JSON(anything=w135) -> (JSON string=w131:string)  [unwired: 2 in, 1 out]
      n62 = Format Into String(format string="\"%s\":%s," ("格式字符串"), w133, w131) -> (resulting string=w132:string)  [unwired: 2 in, 1 out]
    }
  }
  n63 = case shown="True" w25 {
    tunnel: w24 -> [_ w140]
    tunnel: w23 -> [_ w138]
    tunnel: [_ w137] -> w4
    frame False {
    }
    frame True {
      n64 = Flatten To JSON(anything=w140) -> (JSON string=w136:string)  [unwired: 2 in, 1 out]
      n65 = Format Into String(format string="\"%s\":%s," ("格式字符串"), w138, w136) -> (resulting string=w137:string)  [unwired: 2 in, 1 out]
    }
  }
  n66 = case shown="True" w20 {
    tunnel: w21 -> [_ w145]
    tunnel: w22 -> [_ w143]
    tunnel: [_ w142] -> w3
    frame False {
    }
    frame True {
      n67 = Flatten To JSON(anything=w145) -> (JSON string=w141:string)  [unwired: 2 in, 1 out]
      n68 = Format Into String(format string="\"%s\":%s," ("格式字符串"), w143, w141) -> (resulting string=w142:string)  [unwired: 2 in, 1 out]
    }
  }
  n69 = case shown="True" w14 {
    tunnel: w15 -> [_ w150]
    tunnel: w16 -> [_ w148]
    tunnel: [_ w147] -> w2
    frame False {
    }
    frame True {
      n70 = Flatten To JSON(anything=w150) -> (JSON string=w146:string)  [unwired: 2 in, 1 out]
      n71 = Format Into String(format string="\"%s\":%s," ("格式字符串"), w148, w146) -> (resulting string=w147:string)  [unwired: 2 in, 1 out]
    }
  }
  n72 = case shown="True" w19 {
    tunnel: w18 -> [_ w155]
    tunnel: w17 -> [_ w153]
    tunnel: [_ w152] -> w1
    frame False {
    }
    frame True {
      n73 = Flatten To JSON(anything=w155) -> (JSON string=w151:string)  [unwired: 2 in, 1 out]
      n74 = Format Into String(format string="\"%s\":%s," ("格式字符串"), w153, w151) -> (resulting string=w152:string)  [unwired: 2 in, 1 out]
    }
  }
  n75 = Build Array(w41, w40, w39, w38, w37, w36, w35, w34, w5, w4, w3, w2, w1) -> (w33:string[])
  n76 = for {
    tunnel: w45 -> [w174]
    tunnel: w33 -> [w172] mode=indexing
    shift-right: [w169] -> w31
    shift-left: string[] [] ("json") -> [w171]
    n77 = Empty String/Path?(string/path=w172) -> (empty?=w168:bool)
    n78 = case shown="False" w168 {
      tunnel: w172 -> [w184 w185]
      tunnel: [w181 w185] -> w166
      frame False {
        n79 = String Length(string=w184) -> (length=w183:i32)
        n80 = Decrement(x=w183) -> (x-1=w182:i32)
        n81 = String Subset(string=w184, length (rest)=w182) -> (substring=w181:string)  [unwired: 1 in]
      }
      frame True {
      }
    }
    n82 = Search and Replace String(replace all?=TRUE ("替换全部？(F)"), case sensitive?=TRUE ("忽略大小写？(F)"), input string=w166, search string="-Infinity" ("搜索字符串"), replace string="0" ("替换字符串(\"\")")) -> (result string=w158:string, error out=w156:errorcluster)  [unwired: 3 in, 2 out]
    n83 = control-ref of="time"() -> (w173:refnum<vi>)
    n84 = property class="Str"(reference=w173) -> ("Label.Text"=w175:string)  [unwired: 1 in, 2 out]
    n85 = Search and Replace String(replace all?=TRUE ("替换全部？(F)"), case sensitive?=TRUE ("忽略大小写？(F)"), input string=w158, search string="NaN" ("搜索字符串"), replace string="0" ("替换字符串(\"\")"), error in=w156) -> (result string=w157:string)  [unwired: 2 in, 3 out]
    n86 = Format Into String(format string="{\"%s\":\"%s\",\"data\":{%s}}" ("格式字符串"), w175, w174, w157) -> (resulting string=w170:string)  [unwired: 2 in, 1 out]
    n87 = case shown="False" w168 {
      tunnel: w171 -> [w179 w180]
      tunnel: w170 -> [w178 _]
      tunnel: [w177 w180] -> w169
      frame False {
        n88 = Build Array (concatenate)(w179, w178) -> (w177:string[])
      }
      frame True {
      }
    }
  }
  "json" <- w31
